vi "OAT Auto Labeled Polar Plot.vi"(0 "picture":picture, 1 "picture \ndimensions (w,h)":cluster{"width":i16, "height":i16}, 2 "polar settings":T3={"polar attributes"={"maximum"=0.0, "minimum"=0.0, "clip to min"=FALSE, "log"=FALSE, "grid color"=3381657, "plot color"=16711680, "fmt and prec"={"format"=enum."Decimal", "precision"=1}, "visible section"=8}, "desired font(Application)"=enum."Application Font", "[user-specified font]"={"Font Name:"="", "Size"=0, "Strikeout?"=FALSE, "Italic?"=FALSE, "Underline?"=FALSE, "Outline?"=FALSE, "Shadow?"=FALSE, "Bold?"=FALSE}} {"polar attributes"."minimum" format="%.2f"; "polar attributes"."maximum" format="%.2f"}, 3 "cursor attributes":T4={"layout color"=852223, "active color"=16740820, "precision"=2, "BG transparent? (T)"=FALSE, "radius"=2}, 5 "magnitude":cluster{"X":dbl[], "Y":dbl[]} {"Y" format="%.2f"; "X" format="%.2f"}, 7 "phase lag(rad)":cluster{"X":dbl[], "Y":dbl[]} {"Y" format="%.2f"; "X" format="%.2f"}, 11 "error in (no error)":errorcluster, 12 "rotating settings":T2 {"probe position" items=["0", "45", "90", "135", "180", "225", "270", "315"]; "shatft rotating direction" items=["CW", "CCW"]}, 13 "phase setting":T1, 14 "avoid overlap? (Y)":bool=TRUE) -> (4 "new picture":picture, 15 "error out":errorcluster)   [LabVIEW 2017]
doc: "Draws and labels a polar plot on a picture control."
uses:
  <vilib>/addons/Sound and Vibration/Order Analysis/Backward Compatibility/SubVIs/OAT Polar Cursor Attributes.ctl
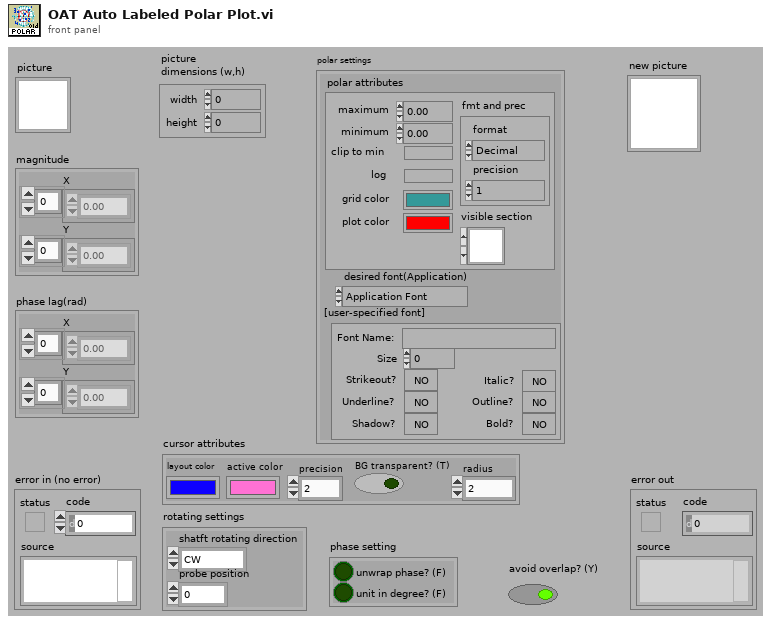
[diagram p1: front panel]
types:
  T1 = cluster{"unwrap phase? (F)":bool, "unit in degree? (F)":bool}
  T2 = cluster{"shatft rotating direction":u16, "probe position":u16}
  T3 = cluster{"polar attributes":cluster{"maximum":dbl, "minimum":dbl, "clip to min":bool, "log":bool, "grid color":u32, "plot color":u32, "fmt and prec":cluster{"format":enum8{"Decimal", "Scientific", "Engineering", "Binary", "Octal", "Hex"}, "precision":u8}, "visible section":u16}, "desired font(Application)":enum16{"User-specified Font", "Application Font", "System Font", "Dialog Font"}, "[user-specified font]":cluster{"Font Name:":string, "Size":i16, "Strikeout?":bool, "Italic?":bool, "Underline?":bool, "Outline?":bool, "Shadow?":bool, "Bold?":bool}}
  T4 = typedef "OAT Polar Cursor Attributes.ctl" = cluster{"layout color":u32, "active color":u32, "precision":i16, "BG transparent? (T)":bool, "radius":i16}
  T5 = cluster{"maximum":dbl, "minimum":dbl, "clip to min":bool, "log":bool, "grid color":u32, "plot color":u32, "fmt and prec":cluster{"format":enum8{"Decimal", "Scientific", "Engineering", "Binary", "Octal", "Hex"}, "precision":u8}, "visible section":u16}
  T6 = cluster{"Name":string, "Location":cluster{"mag":dbl, "phase":dbl}}[]
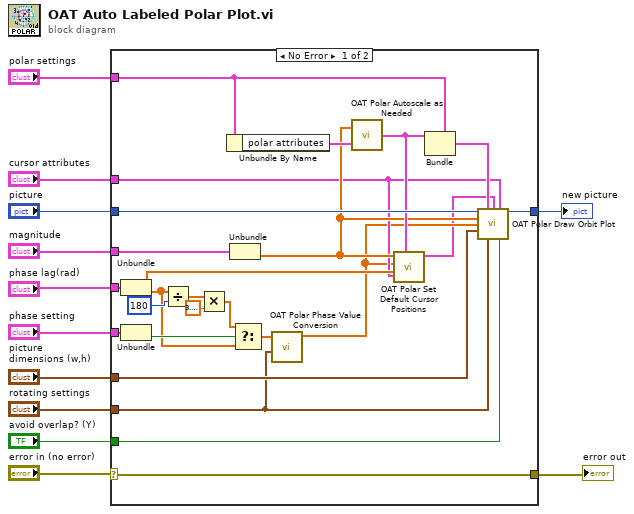
[diagram p0: block diagram]
diagram:
  n1 = case shown="No Error" "error in (no error)" {
    selector: "error in (no error)" -> [w13 w39]
    tunnel: "polar settings" -> [w37 _]
    tunnel: [w36 w38] -> w11
    tunnel: "magnitude" -> [w35 _]
    tunnel: "phase lag(rad)" -> [w34 _]
    tunnel: "avoid overlap? (Y)" -> [w33 _]
    tunnel: "picture" -> [w30 w38]
    tunnel: "cursor attributes" -> [w26 _]
    tunnel: "picture \ndimensions (w,h)" -> [w25 _]
    tunnel: "phase setting" -> [w22 _]
    tunnel: "rotating settings" -> [w14 _]
    tunnel: [w13 w39] -> w1
    frame No Error {
      n2 = Unbundle(w34) -> ("X"=w28:dbl[], "Y"=w16:dbl[])
      n3 = Unbundle(w22) -> ("unit in degree? (F)"=w21:bool)  [unwired: 1 out]
      n4 = Divide(x=w16, y=180) -> (x/y=w19:dbl[])
      n5 = Multiply(x=w19, y=3.141592653589793) -> (x*y=w17:dbl[])
      n6 = Unbundle By Name(w37) -> ("polar attributes"=w31:T5)
      n7 = Unbundle(w35) -> ("Y"=w27:dbl[])  [unwired: 1 out]
      n8 = Select(t=w17, s=w21, f=w16) -> (s? t:f=w15:dbl[])
      n9 = call <vilib>:"OAT Polar Phase Value Conversion.vi"("channel settings"=w14, "phases in"=w15) -> ("phases out"=w24:dbl[])  [unwired: 9 in]
      n10 = call <vilib>:"OAT Polar Autoscale as Needed.vi"("polar attributes"=w31, "magnitudes (even angular)"=w27) -> ("polar attributes"=w29:T5)
      n11 = call <vilib>:"OAT Polar Set Default Cursor Positions.vi"("cursor attributes"=w26, "polar attributes"=w29, "cursor values"=w28, "phases"=w24, "magnitudes (even angular)"=w27) -> ("Cursor List (EU position]"=w23:T6)  [unwired: 6 in]
      n12 = Bundle(cluster=w37, "polar attributes"=w29) -> (w32:T3)  [unwired: 2 in]
      n13 = call <vilib>:"OAT Polar Draw Orbit Plot.vi"("picture"=w30, "polar settings"=w32, "Cursor List (EU position]"=w23, "cursor attributes"=w26, "magnitudes (even angular)"=w27, "phases"=w24, "picture \ndimensions (w,h)"=w25, "channel settings"=w14, "avoid overlap? (Y)"=w33) -> ("picture out"=w36:picture)  [unwired: 5 in, 1 out]
    }
    frame Error {
    }
  }
  "new picture" <- w11
  "error out" <- w1
